vi "comb-YangZhang.vi"(0 "fs":dbl, 2 "f1":dbl, 3 "f2":dbl, 5 "R":dbl) -> (1 "reverse coefficients":dbl[](array[numeric]), 4 "foward coefficients":dbl[](array[numeric]), 6 "Magnitude":cluster{dbl[], dbl[]}(graph), 7 "Phase":cluster{dbl[], dbl[]}(graph), 8 "Pole-Zero Plot":cluster{dbl[], dbl[]}[](graph))   [LabVIEW 2016]
uses:
  <vilib>/imath/engines/lvmath2/RunTimeEngine/Managers/WorkSpace/UID Generator.vi
  <vilib>/imath/engines/lvmath2/RunTimeEngine/BuiltInFunctions/conv/NIMS_conv(V,V).vi
  <instcachedir>/0/NIMS_conv(V,V)_D3E194F2B5174935BB2368CEB7AAC5A9.lvgen/NIMS_conv(V,V)_D3E194F2B5174935BB2368CEB7AAC5A9_000.vi
  <vilib>/imath/engines/lvmath2/RunTimeEngine/RunTimeType/NIMS_RunTimeType_From StrictType (excl LVString).vi
  <instcachedir>/0/NIMS_RunTimeType_From StrictType (excl LVString)_BBF44FB49F834B71AF7A14CCEDF8BECD.lvgen/NIMS_RunTimeType_From StrictType (excl LVString)_BBF44FB49F834B71AF7A14CCEDF8BECD_000.vi
  <vilib>/imath/engines/lvmath2/RunTimeEngine/ErrorHandling/NIMS_Error From Error Code.vi
  <vilib>/imath/engines/lvmath2/RunTimeEngine/LocalVariableDefStatement/MC_LocalVariableDefStatement_Display.vi
  <vilib>/imath/engines/lvmath2/RunTimeEngine/Managers/SymbolTable/Clear UID.vi
  <vilib>/imath/engines/lvmath2/RunTimeEngine/NodeEndStatement/NIMS_NodeEndStatement_Output.vi
  <instcachedir>/0/NIMS_NodeEndStatement_Output_53EC0D466D134D7ABD903AC30B43404B.lvgen/NIMS_NodeEndStatement_Output_53EC0D466D134D7ABD903AC30B43404B_005.vi
  <vilib>/imath/engines/lvmath2/RunTimeEngine/ErrorHandling/NIMS_Finalize Error.vi
  Program Files (x86)/National Instruments/Scripts/Plot Frequency Response - direct.vi
  Program Files (x86)/National Instruments/Scripts/Plot Pole-Zero - direct.vi
  <vilib>/imath/engines/lvmath2/RunTimeEngine/Managers/SymbolTable/NIMS_WorkSpace.lvlib
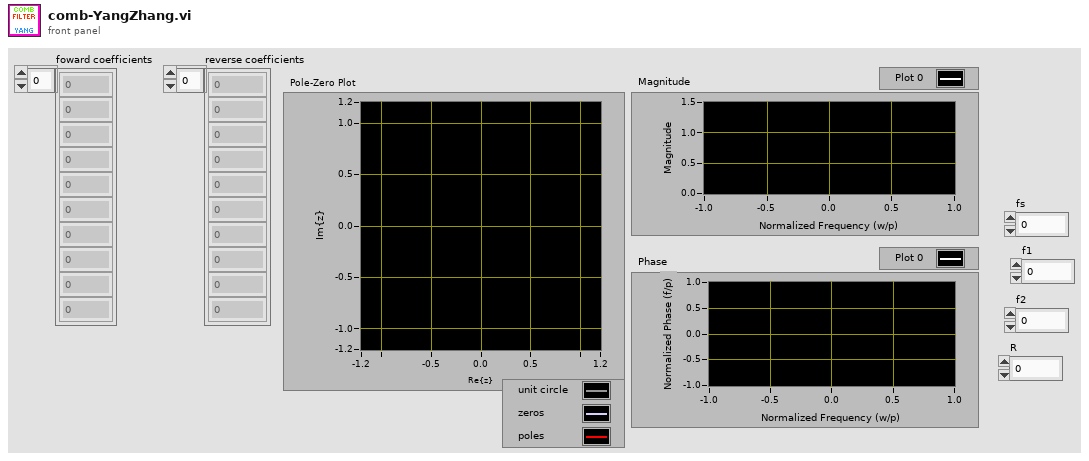
[diagram p1: front panel]
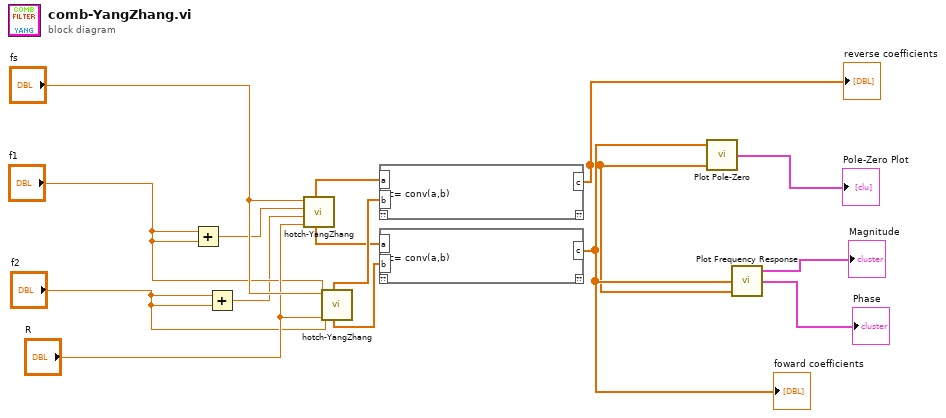
[diagram p0: block diagram]
diagram:
  n1 = Add(x="f1", y="f1") -> (x+y=w13:dbl)
  n2 = Add(x="f2", y="f2") -> (x+y=w11:dbl)
  n3 = call "hotch-YangZhang.vi"("fs"="fs", "f1"=w13, "f2"=w11, "R"="R") -> ("reverse coefficients"=w9:dbl[], "forward coefficients"=w7:dbl[])  [unwired: 3 out]
  n4 = call "hotch-YangZhang.vi"("fs"="fs", "f1"="f1", "f2"="f2", "R"="R") -> ("reverse coefficients"=w8:dbl[], "forward coefficients"=w6:dbl[])  [unwired: 3 out]
  n5 = mathscript code="c= conv(a,b)"("a"=w9, "b"=w8) -> ("c"=w1:dbl[])  [unwired: 1 in, 1 out]
  "reverse coefficients" <- w1
  n6 = mathscript code="c= conv(a,b)"("a"=w7, "b"=w6) -> ("c"=w2:dbl[])  [unwired: 1 in, 1 out]
  "foward coefficients" <- w2
  n7 = call-poly "Plot Pole-Zero.vi"("a, reverse coefficients"=w1, "b, forward coefficients"=w2) -> ("Pole-Zero Plot"=→"Pole-Zero Plot":cluster{dbl[], dbl[]}[])  [unwired: 3 in]
  n8 = call-poly "Plot Frequency Response.vi"("b, forward coefficients"=w2, "a, reverse coefficients"=w1) -> ("Magnitude"=→"Magnitude":cluster{dbl[], dbl[]}, "Phase"=→"Phase":cluster{dbl[], dbl[]})  [unwired: 3 in, 1 out]
